vi "MCCETC02_Main.vi"() -> ()   [LabVIEW 2019]
panel:
  out "T6":dbl format="%.2f"
  out "T5":dbl format="%.2f"
  out "T4":dbl format="%.2f"
  out "T3":dbl format="%.2f"
  out "T2":dbl format="%.2f"
  in  "Tab Control":enum32{"IVC & Fridge", "Microwave System"}(tab)
  out "T0 Chart":waveform(dbl)[](graph)
  out "T1 Chart":waveform(dbl)[](graph)
  out "T2 Chart":waveform(dbl)[](graph)
  out "T3 Chart":waveform(dbl)[](graph)
  out "T4 Chart":waveform(dbl)[](graph)
  out "T5 Chart":waveform(dbl)[](graph)
  out "T6 Chart":waveform(dbl)[](graph)
  in  "Readout Interval":i32=5 caption="sec"
  in  "units":i32(ring) items=["degC", "degF", "kelvin", "raw"]
  out "T1":dbl format="%.2f"
  out "T0":dbl format="%.2f"
  out "Readout Status":bool
  out "Last Measured":timestamp format="%<%Y-%m-%d %H:%M:%S>T"
  in  "Stop":bool
  # "MCC E-TC #02"
  # "IVC Bottom"
  # "IVC Top"
  # "Fridge Top"
  # "LHe FL Stinger"
  # "LHe FL #1"
  # "LHe FL #2"
  # "Sep. Line"
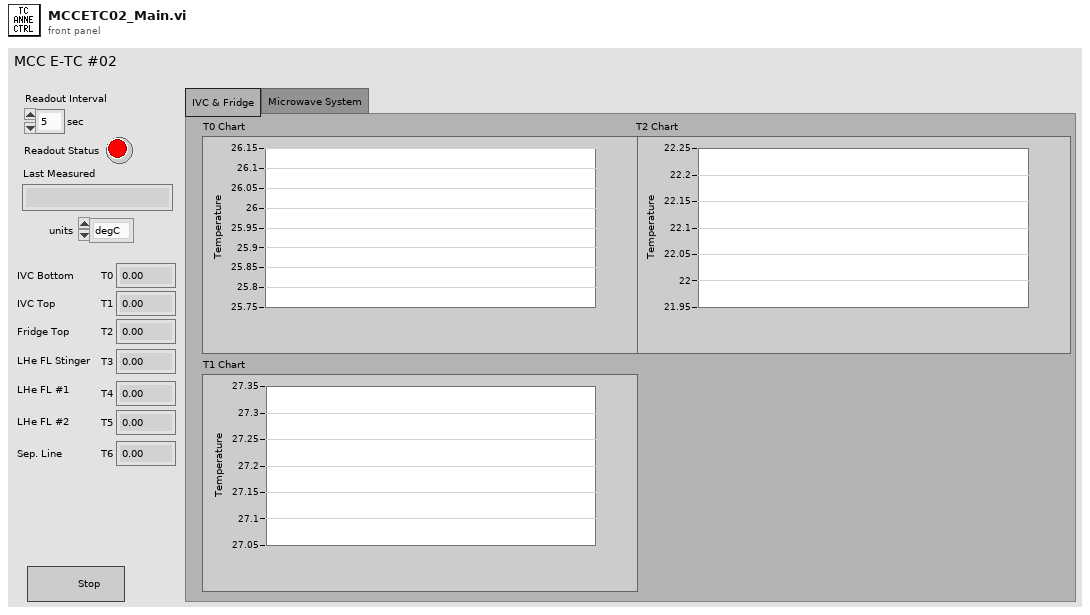
[diagram p1: front panel]
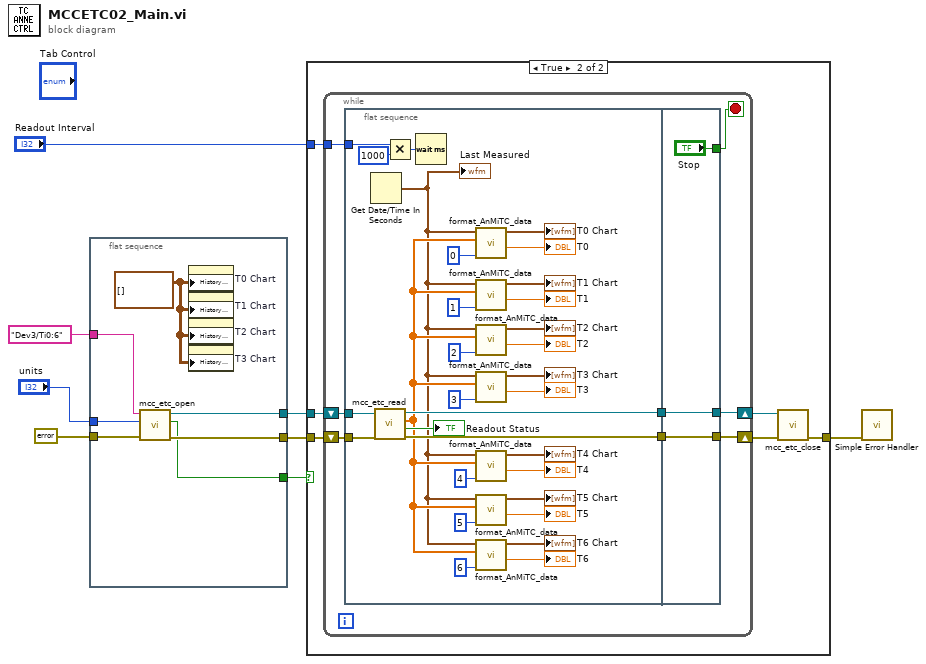
[diagram p0: block diagram]
diagram:
  n1 = flat-sequence {
    tunnel: [w15] -> w8
    tunnel: errorcluster {"status"=FALSE, "code"=0, "source"=""} ("error in") -> [w14]
    tunnel: [w13] -> w6
    tunnel: "Dev3/Ti0:6" ("Device/Channel Name") -> [w12]
    tunnel: "units" -> [w11]
    tunnel: [w9] -> w1
    frame #0 {
      w10 = waveform(dbl)[][] [] ("History Data")
      n2 = call "mcc_etc_open.vi"("error in"=w14, "units"=w11, "name"=w12) -> ("error out"=w13:errorcluster, "status"=w9:bool, "task out"=w15:refnum<k24>)  [unwired: 6 in]
      n3 = property on="T0 Chart" class="WFChart (strict)"("History Data"=w10) -> ()  [unwired: 2 in, 2 out]
      n4 = property on="T1 Chart" class="WFChart (strict)"("History Data"=w10) -> ()  [unwired: 2 in, 2 out]
      n5 = property on="T2 Chart" class="WFChart (strict)"("History Data"=w10) -> ()  [unwired: 2 in, 2 out]
      n6 = property on="T3 Chart" class="WFChart (strict)"("History Data"=w10) -> ()  [unwired: 2 in, 2 out]
    }
  }
  n7 = case shown="True" w1 {
    tunnel: w8 -> [_ w22]
    tunnel: w6 -> [w16 w21]
    tunnel: "Readout Interval" -> [_ w18]
    tunnel: [w16 w17] -> w2
    frame False {
    }
    frame True {
      n8 = while {
        shift-right: [w28] -> w19
        shift-left: w21 -> [w29]
        shift-right: [w27] -> w20
        shift-left: w22 -> [w30]
        tunnel: w18 -> [w26]
        stop <- w23 stop-if-true
        n9 = flat-sequence {
          tunnel: w30 -> [w61]
          tunnel: w29 -> [w60]
          tunnel: w26 -> [w56]
          tunnel: [w59] -> w25
          tunnel: [w58] -> w24
          tunnel: [w63] -> w27
          tunnel: [w64] -> w28
          tunnel: w25 -> [w64]
          tunnel: w24 -> [w63]
          tunnel: ["Stop"] -> w23
          frame #0 {
            n10 = Get Date/Time In Seconds() -> (seconds since 1Jan1904=w37:timestamp)
            "Last Measured" <- w37
            n11 = call "mcc_etc_read.vi"("error in"=w60, "task in"=w61) -> ("error out"=w59:errorcluster, "status"=→"Readout Status":bool, "temperature_array"=w38:dbl[], "task out"=w58:refnum<k24>)  [unwired: 6 in]
            n12 = Multiply(x=w56, y=1000) -> (x*y=w43:i32)
            n13 = Wait (ms)(milliseconds to wait=w43) -> ()  [unwired: 1 out]
            n14 = call "format_AnMiTC_data.vi"("index"=0, "value_array"=w38, "time"=w37) -> ("value"=→"T0":dbl, "waveform_array"=→"T0 Chart":waveform(dbl)[])  [unwired: 7 in]
            n15 = call "format_AnMiTC_data.vi"("index"=1, "value_array"=w38, "time"=w37) -> ("value"=→"T1":dbl, "waveform_array"=→"T1 Chart":waveform(dbl)[])  [unwired: 7 in]
            n16 = call "format_AnMiTC_data.vi"("index"=2, "value_array"=w38, "time"=w37) -> ("value"=→"T2":dbl, "waveform_array"=→"T2 Chart":waveform(dbl)[])  [unwired: 7 in]
            n17 = call "format_AnMiTC_data.vi"("index"=3, "value_array"=w38, "time"=w37) -> ("value"=→"T3":dbl, "waveform_array"=→"T3 Chart":waveform(dbl)[])  [unwired: 7 in]
            n18 = call "format_AnMiTC_data.vi"("index"=4, "value_array"=w38, "time"=w37) -> ("value"=→"T4":dbl, "waveform_array"=→"T4 Chart":waveform(dbl)[])  [unwired: 7 in]
            n19 = call "format_AnMiTC_data.vi"("index"=5, "value_array"=w38, "time"=w37) -> ("value"=→"T5":dbl, "waveform_array"=→"T5 Chart":waveform(dbl)[])  [unwired: 7 in]
            n20 = call "format_AnMiTC_data.vi"("index"=6, "value_array"=w38, "time"=w37) -> ("value"=→"T6":dbl, "waveform_array"=→"T6 Chart":waveform(dbl)[])  [unwired: 7 in]
          }
          frame #1 {
          }
        }
      }
      n21 = call "mcc_etc_close.vi"("error in"=w19, "task in"=w20) -> ("error out"=w17:errorcluster)  [unwired: 8 in, 1 out]
    }
  }
  n22 = call <vilib>:"Simple Error Handler.vi"("error in (no error)"=w2) -> ()  [unwired: 4 in, 5 out]
